vi "Error Handler.vi"(8 "error in (no error)":errorcluster, 9 "handle warnings? (F)":bool, 10 "dialog? (T)":bool=TRUE) -> (0 "error out":errorcluster, 2 "error text":string)   [LabVIEW 2018, in "STEPkgDriver_LINC.lvlib"]
uses:
  STEPkgDriver_LINC.lvlib
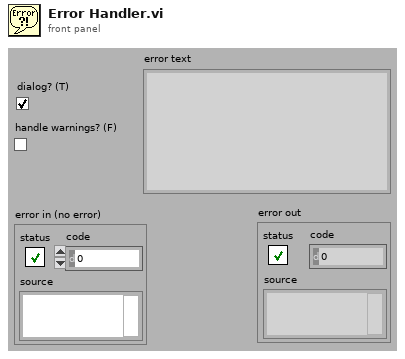
[diagram p1: front panel]
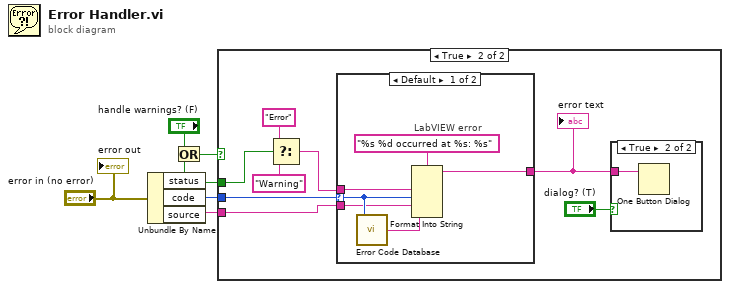
[diagram p0: block diagram]
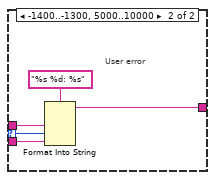
[diagram p4: hidden frame]
diagram:
  n1 = Unbundle By Name("error in (no error)") -> ("status"=w1:bool, "code"=w3:i32, "source"=w2:string)
  n2 = Or(x="handle warnings? (F)", y=w1) -> (x .or. y?=w4:bool)
  n3 = case shown="True" w4 {
    tunnel: w3 -> [_ w12]
    tunnel: w2 -> [_ w11]
    tunnel: w1 -> [_ w10]
    frame False {
    }
    frame True {
      n4 = Select(t="Error", s=w10, f="Warning") -> (s? t:f=w7:string)
      n5 = case shown="Default" w12 {
        selector: w12 -> [w20 w26]
        tunnel: w11 -> [w19 w25]
        tunnel: [w17 w23] -> w14
        tunnel: w7 -> [w16 w22]
        frame Default {
          # "LabVIEW error"
          n6 = call <vilib>:"Error Code Database.vi"("Error Code"=w20) -> ("Error Text"=w18:string)
          n7 = Format Into String(format string="%s %d occurred at %s: %s", w16, w20, w19, w18) -> (resulting string=w17:string)  [unwired: 2 in, 1 out]
        }
        frame -1400..-1300, 5000..10000 {
          # "User error"
          n8 = Format Into String(format string="%s %d: %s", w22, w26, w25) -> (resulting string=w23:string)  [unwired: 2 in, 1 out]
        }
      }
      "error text" <- w14
      n9 = case shown="True" "dialog? (T)" {
        tunnel: w14 -> [_ w15]
        frame False {
        }
        frame True {
          n10 = One Button Dialog(message=w15) -> ()  [unwired: 1 in, 1 out]
        }
      }
    }
  }
  "error out" <- "error in (no error)"
